vi "String Name Display.vi"() -> ()   [LabVIEW 2015]
panel:
  in  "stop":bool
  in  "String":string
  out "concatenated string":string
  # "Name Display"
  # "Pardeep Kumar"
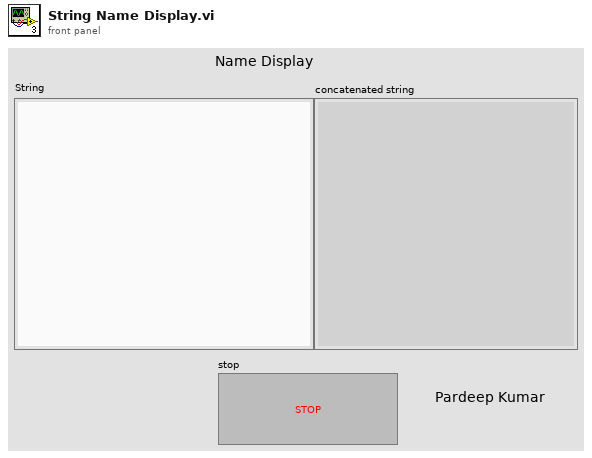
[diagram p1: front panel]
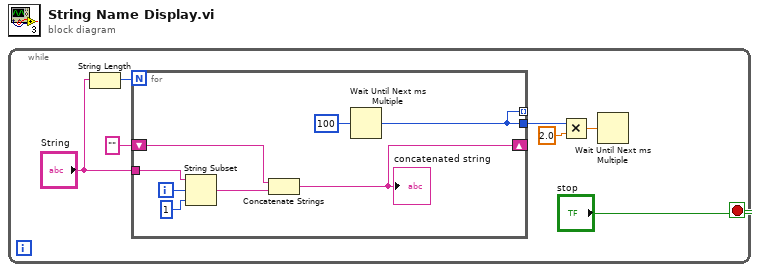
[diagram p0: block diagram]
diagram:
  n1 = while {
    stop <- "stop" stop-if-true
    n2 = String Length(string="String") -> (length=w7:i32)
    n3 = for {
      N: w7 -> [_]
      tunnel: "String" -> [w15]
      shift-right: [w11] -> _
      shift-left: "" -> [w10]
      tunnel: [w8] -> w4
      tunnel: [w8] -> _ mode=indexing
      i -> [w14]
      n4 = String Subset(string=w15, offset (0)=w14, length (rest)=1 ("length (rest)")) -> (substring=w12:string)
      n5 = Concatenate Strings "Concatenate Strings"(w10, w12) -> (w11:string)
      "concatenated string" <- w11
      n6 = Wait Until Next ms Multiple(millisecond multiple=u32 100) -> (millisecond timer value=w8:u32)
    }
    n7 = Multiply(x=w4, y=2.0) -> (x*y=w3:dbl)
    n8 = Wait Until Next ms Multiple(millisecond multiple=w3) -> ()  [unwired: 1 out]
  }
